vi "7.0-Global.vi"() -> ()   [LabVIEW 2011]
uses:
  4-High Neurons/4.0-Timing Badass.ctl
  6-OCU Neurons/6.1-Act.ctl
  6-OCU Neurons/6.1-UDP Saitek.ctl
  7.0-OCU State.ctl
  7.0 GUI/7.0 Auto Mode Display.ctl
  <vilib>/robotics/Controls/Compass Indicator/Compass Indicator.xctl
  7.0 GUI/7.0 Manual Mode Display.ctl
  6-OCU Neurons/6.3-What Reporting.ctl
  6-OCU Neurons/6.3-Lidar Data.ctl
  6-OCU Neurons/6.4-How Reporting Typedef.ctl
  7.0 GUI/7.0 Manual Mode Buttons.ctl
  7.0 GUI/7.0 Auto Mode Buttons.ctl
  4-High Neurons/4.2-Where Sensor Typedef.ctl
  4-High Neurons/Current GPS Data.ctl
  3-Midbrain/3.2-Where/_typedefs/3.2.1-VectorNav Data.ctl
  7.3-Mission Def/7.6 - GPS Waypoint Def.ctl
  6-OCU Neurons/MDF Array LatLong.ctl
  6-OCU Neurons/MDF LatLong.ctl
  4-High Neurons/4.2/4.2.0 Kalman State.ctl
panel:
  in  "7.0 GUI Tab Equivalent State":T1
  in  "GUI shutdown Button":bool
  in  "7.0 OCU State":T1
  in  "Manual Override":bool
  in  "Stop Loops":bool
  in  "Main Tab Interface":T2(tab)
  in  "7.1-Act Resolution":sgl=91.0
  in  "6.1 Act":T3 {"6.1-Saitek Controller"."Right" scale=0.0..1.0; "6.1-Saitek Controller"."Left" scale=0.0..1.0; "6.1-Saitek Controller"."Yaw" scale=-1.0..1.0; "6.1-Saitek Controller"."Roll" scale=-1.0..1.0; "6.1-Saitek Controller"."Pitch" scale=-1.0..1.0}
  out "7.2-Where Am I? Sensor":T5 {"4.2.2- Current GPS Data"."Longitude (Decimal Degrees)" format="%#.6g"; "4.2.2- Current GPS Data"."Lattitude (Decimal Degrees)" format="%#.6g"}
  out "7.2 -State Vector X":T8
  in  "4.3-What":T9
  in  "6.4 How":T11
  in  "7.6 - Current Waypoint":T12
  out "7.6 - Has Mission Def":bool
  in  "7.6 - GPS Waypoints Data":T13={"GPS Waypoint Center (Lat, Long)"=[42.2942563565636, -71.264449], "5.1.1 MDF GPS"=[{"Waypoint #"=0.0, "Latitude (waypoint)"=42.29384665383309, "Longitude  (waypoint)"=-71.264884695410730002}, {"Waypoint #"=1.0, "Latitude (waypoint)"=42.294025217094160001, "Longitude  (waypoint)"=-71.26461245119572}, {"Waypoint #"=2.0, "Latitude (waypoint)"=42.294031169194135002, "Longitude  (waypoint)"=-71.26444883644581}, {"Waypoint #"=3.0, "Latitude (waypoint)"=42.294193859709174999, "Longitude  (waypoint)"=-71.264368370175360003}, {"Waypoint #"=4.0, "Latitude (waypoint)"=42.294256356563590001, "Longitude  (waypoint)"=-71.26427851617336}]} {"5.1.1 MDF GPS"."Latitude (waypoint)" format="%#_8g"; "5.1.1 MDF GPS"."Longitude  (waypoint)" format="%#_8g"}
  in  "7.0 Start Time":dbl
  out "7.0-Manual Mode Controls":T16
  out "7.0 Manual Mode":T17 {"Speed (m/s)" scale=0.0..2.5; "Battery" scale=22.0..24.0; "6.1-Saitek Controller"."Right" scale=0.0..1.0; "6.1-Saitek Controller"."Left" scale=0.0..1.0; "6.1-Saitek Controller"."Yaw" scale=-1.0..1.0; "6.1-Saitek Controller"."Roll" scale=-1.0..1.0; "6.1-Saitek Controller"."Pitch" scale=-1.0..1.0}
  out "7.0 Auto Mode Controls":T18
  out "7.0 Auto Mode Display":T19 {"Speed (m/s)" scale=0.0..2.5; "Battery" scale=20.0..24.0}
  in  "6.7.4 How UDP Period":u32=50
  in  "6.7.3 What TCP Period":u32=50
  in  "6.7.2 Where UDP Period":u32=50
  in  "6.7.1 Act TCP Period":u32=50
  in  "6.7.1 Act UDP Period":u32=50
  in  "6.7.1 Act TCP Server Error":errorcluster
  out "6.7.1 Act TCP Server HB":T20
  in  "6.7.1 Act UDP Server Error":errorcluster
  in  "6.7.2 Where UDP Client Error":errorcluster
  in  "6.7.3 What TCP Client Error":errorcluster
  in  "6.7.4 How UDP Client Error":errorcluster
  out "6.7.1 Act UDP Server HB":T20
  out "6.7.2 Where UDP Client HB":T20
  out "6.7.3 What TCP Client HB":T20
  out "6.7.4 How UDP Client HB":T20
  out "7.8 GUI Loop Timing":T20
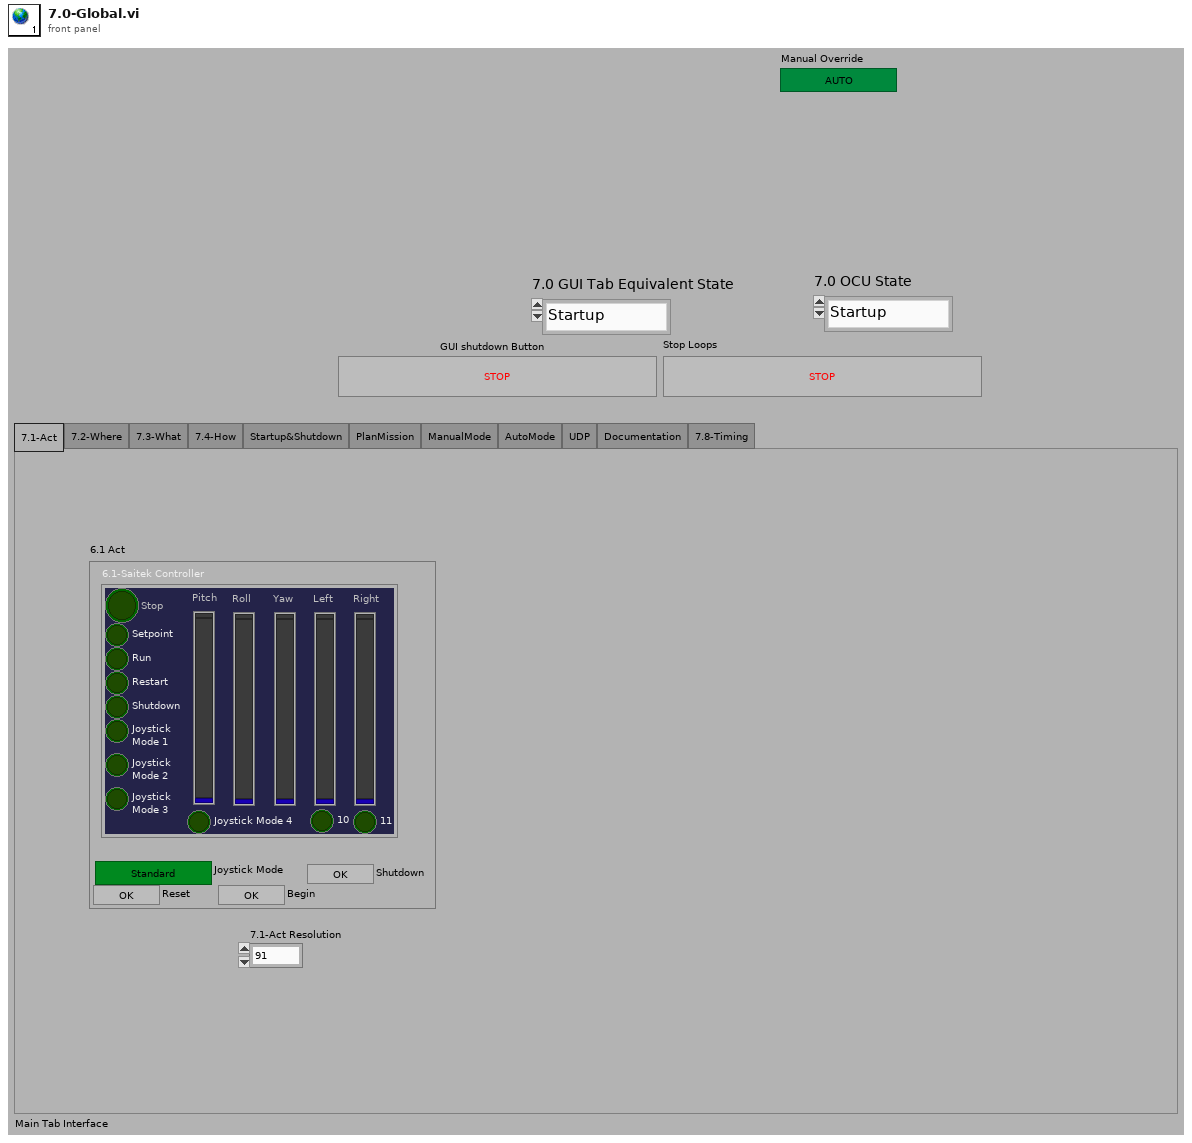
[diagram p1: front panel]
types:
  T1 = typedef "7.0-OCU State.ctl" = enum16{"Startup", "Self Test", "Manual Mode", "Auto Mode", "Plan Mission", "Shutdown"}
  T2 = enum32{"7.1-Act", "7.2-Where", "7.3-What", "7.4-How", "Startup&Shutdown", "PlanMission", "ManualMode", "AutoMode", "UDP", "Documentation", "7.8-Timing"}
  T3 = typedef "6.1-Act.ctl" = cluster{"6.1-Saitek Controller":T4, "Joystick Mode":bool, "Shutdown":bool, "Reset":bool, "Begin":bool}
  T4 = typedef "6.1-UDP Saitek.ctl" = cluster{"Stop":bool, "Setpoint":bool, "Run":bool, "Restart":bool, "Shutdown":bool, "Joystick\nMode 1":bool, "Joystick\nMode 2":bool, "Joystick \nMode 3":bool, "Joystick Mode 4":bool, "10":bool, "11":bool, "Pitch":sgl, "Roll":sgl, "Yaw":sgl, "Left":sgl, "Right":sgl}
  T5 = typedef "4.2-Where Sensor Typedef.ctl" = cluster{"4.2.2- Current GPS Data":T6, "4.2.1-VectorNav Data":T7, "4.2.1-VectorNav Status":string}
  T6 = typedef "Current GPS Data.ctl" = cluster{"Lattitude (Decimal Degrees)":ext, "Longitude (Decimal Degrees)":ext, "EST Time":timestamp}
  T7 = typedef "3.2.1-VectorNav Data.ctl" = cluster{"Yaw":dbl, "Pitch":dbl, "Roll":dbl}
  T8 = typedef "4.2.0 Kalman State.ctl" = cluster{"X":dbl, "Y":dbl, "Theta":dbl, "V":dbl, "Omega":dbl, "Omega Dot":dbl}
  T9 = typedef "6.3-What Reporting.ctl" = cluster{"Local Map":dbl[][], "6.7-Lidar Data":T10}
  T10 = typedef "6.3-Lidar Data.ctl" = cluster{"Angle Array":dbl[], "Magnitude Array":dbl[]}
  T11 = typedef "6.4-How Reporting Typedef.ctl" = cluster{"Drive Speed (m/s)":dbl, "Lidar Inclination (deg) ":dbl, "Steering Angle (deg)":dbl, "Battery Voltage":dbl, "Drive Encoder Cable Check":bool, "Lidar Drive Encoder Cable Check":bool, "Steer Encoder Cable Check":bool, "Lidar Pos Encoder Cable Check":bool, "Mod Buttons & Blinky Cable Check":bool, "Lidar Data Cable Check":bool, "Drive Motor Cable Check":bool, "Vector Nav Cable Check":bool, "Lidar Drive Cable Check":bool, "Steer Drive Cable Check":bool, "Reverse?":bool, "Steering Control Voltage":dbl, "Drive Control Voltage":dbl, "Lidar Control Voltage":dbl}
  T12 = cluster{"Waypoint #":dbl, "X (waypoint)":ext, "Y  (waypoint)":ext}
  T13 = typedef "7.6 - GPS Waypoint Def.ctl" = cluster{"GPS Waypoint Center (Lat, Long)":dbl[], "5.1.1 MDF GPS":T14}
  T14 = typedef "MDF Array LatLong.ctl" = T15[]
  T15 = typedef "MDF LatLong.ctl" = cluster{"Waypoint #":dbl, "Latitude (waypoint)":ext, "Longitude  (waypoint)":ext}
  T16 = typedef "7.0 Manual Mode Buttons.ctl" = cluster{"Joystick Mode":bool, "Reset":bool, "Begin":bool}
  T17 = typedef "7.0 Manual Mode Display.ctl" = cluster{"6.1-Saitek Controller":T4, "Time":dbl, "Battery":dbl, "Speed (m/s)":dbl, "Heading":dbl}
  T18 = typedef "7.0 Auto Mode Buttons.ctl" = cluster{"Enable Joystick":bool, "End Run":bool, "Begin":bool, "Send Map":bool}
  T19 = typedef "7.0 Auto Mode Display.ctl" = cluster{"Shutdown CMD":bool, "Time":dbl, "Battery":dbl, "Speed (m/s)":dbl, "Heading":dbl, "Latitude":dbl, "Longitude":dbl, "Lattitude of Waypoint":dbl, "Longitude of Waypoint":dbl, "Distance to Waypoint (m)":dbl, "Has Mission Def":bool, "XY Graph":cluster{i32[], "Speed By Path":dbl[]}[]}
  T20 = typedef "4.0-Timing Badass.ctl" = cluster{"Loop Period (ms)":u32, "HB":bool, "Last Time (ms)":u32, "Execution (ms)":u32}
diagram:
